vi "create_standardized_delay_array.vi"(4 "delay array":dbl[](array[numeric]), 5 "resolution":i32=100) -> (1 "standardize array":dbl[](array[numeric]), 2 "multiplier":i32)   [LabVIEW 2011]
doc: "creates a standardize array that can be easily displayed no matter what the time unit in the array is. covers second to nanoseconds."
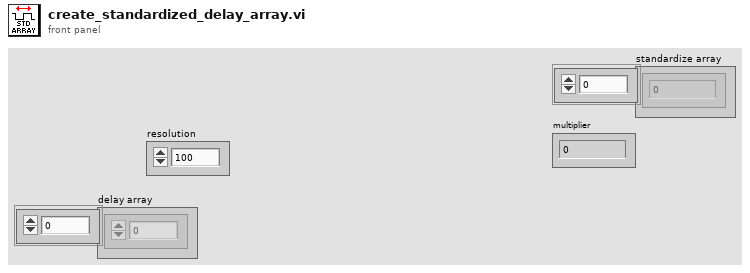
[diagram p1: front panel]
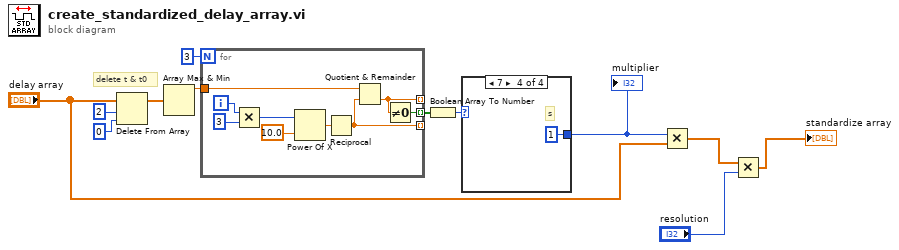
[diagram p0: block diagram]
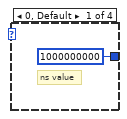
[diagram p2: hidden frame]
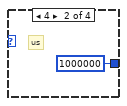
[diagram p3: hidden frame]
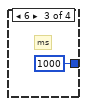
[diagram p4: hidden frame]
diagram:
  # "delete t & t0"
  n1 = Delete From Array(array="delay array", length=2, index=0) -> (array with subset deleted=w7:dbl[])  [unwired: 1 out]
  n2 = Array Max & Min(array=w7) -> (max value=w6:dbl)  [unwired: 3 out]
  n3 = for {
    N: 3 -> [_]
    tunnel: w6 -> [w18]
    tunnel: [w13] -> _ mode=indexing
    tunnel: [w17] -> _ mode=indexing
    tunnel: [w16] -> w11 mode=indexing
    i -> [w15]
    n4 = Multiply(x=w15, y=3) -> (x*y=w19:i32)
    n5 = Power Of X(1:10.0 ("x"), 2:w19) -> (0:w14:dbl)
    n6 = Reciprocal(x=w14) -> (1/x=w13:dbl)
    n7 = Quotient & Remainder(x=w18, y=w13) -> (floor(x/y)=w17:dbl)  [unwired: 1 out]
    n8 = Not Equal To 0?(x=w17) -> (x != 0?=w16:bool)
  }
  n9 = Boolean Array To Number(Boolean array=w11) -> (number=w10:u32)
  n10 = case shown="7" w10 {
    tunnel: [1000000000 1000000 1000 1] -> w5
    frame 0, Default {
      # "ns value"
    }
    frame 4 {
      # "us"
    }
    frame 6 {
      # "ms"
    }
    frame 7 {
      # "s"
    }
  }
  "multiplier" <- w5
  n11 = Multiply(x=w5, y="delay array") -> (x*y=w2:dbl[])
  n12 = Multiply(x=w2, y="resolution") -> (x*y=→"standardize array":dbl[])
